vi "__IFBOX_BPF_CONT2.vi"(0 "YIG frq(GHz) 2":dbl=4.0, 2 "フィルター（1:YIG,2:direct,3:4-12BPF,4:direct4-12BPF）":i16=1, 3 "Dev#":i16) -> ()   [LabVIEW 2017]
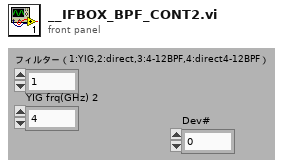
[diagram p1: front panel]
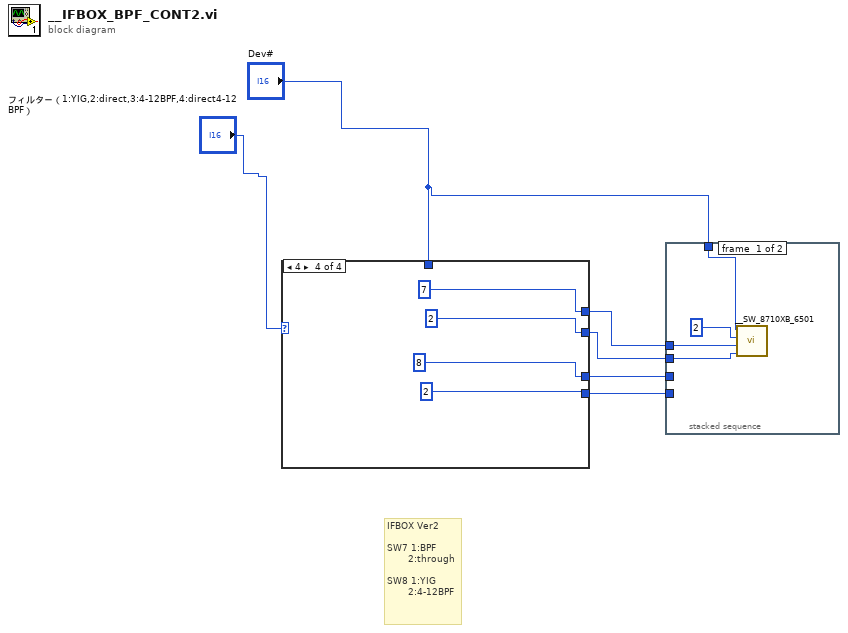
[diagram p0: block diagram]
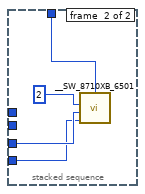
[diagram p2: hidden frame]
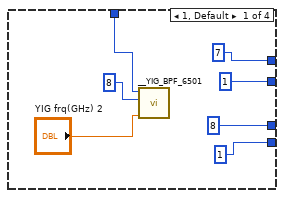
[diagram p3: hidden frame]
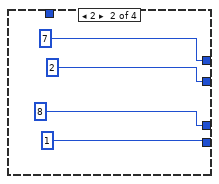
[diagram p4: hidden frame]
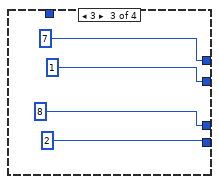
[diagram p5: hidden frame]
diagram:
  # "IFBOX Ver2\n\nSW7 1:BPF\n       2:through\n\nSW8 1:YIG\n       2:4-12BPF"
  n1 = case shown="4" "フィルター（1:YIG,2:direct,3:4-12BPF,4:direct4-12BPF）" {
    tunnel: "Dev#" -> [w11 _ _ _]
    tunnel: [7 7 7 7] -> w5
    tunnel: [1 2 1 2] -> w4
    tunnel: [8 8 8 8] -> w3
    tunnel: [1 1 2 2] -> w2
    frame 1, Default {
      n2 = call "__YIG_BPF_6501.vi"("fc(GHz)"="YIG frq(GHz) 2", "bit"=8, "Dev(1,2..)"=w11) -> ()  [unwired: 1 in]
    }
    frame 2 {
    }
    frame 3 {
    }
    frame 4 {
    }
  }
  n3 = stacked-sequence {
    tunnel: w5 -> [w28 _]
    tunnel: w4 -> [w27 _]
    tunnel: w3 -> [_ w32]
    tunnel: w2 -> [_ w31]
    tunnel: "Dev#" -> [w26 w30]
    frame #0 {
      n4 = call "__SW_8710XB_6501.vi"("Path(1..6)"=w27, "ch(1..6)"=w28, "bit(4or6)"=2, "Dev(1,2..)"=w26) -> ()
    }
    frame #1 {
      n5 = call "__SW_8710XB_6501.vi"("Path(1..6)"=w31, "ch(1..6)"=w32, "bit(4or6)"=2, "Dev(1,2..)"=w30) -> ()
    }
  }
